vi "Load Engine Settings.vi"(8 "error in (no error)":errorcluster, 11 "Device Ref in":T1 format="%.0x") -> (0 "error out":errorcluster, 1 "FIFO Ref out":refnum<k20>, 2 "FPGA Ref out":refnum<k20>, 3 "Device Ref out":T1 format="%.0x")   [LabVIEW 2014, in "SLSC configuration Engine.lvlib"]
uses:
  SLSC configuration Engine.lvlib
  <vilib>/NI Veristand/Custom Device API/Custom Device Item Ref.ctl
  Shared/Type Defs/Device Settings.ctl
  <vilib>/NI/LVFPGA Adv Session Resources/OpenByNameSubVI.vi
  Shared/Constants.vi
  <vilib>/NI Veristand/Custom Device API/Get Item Property (Variant).vi
  <vilib>/FPGAPlugInAG/Dynamic/niLvFpga_Run_Dynamic.vi
  <vilib>/rvi/interface/common/dynamic/niFpgaEscapeDelimiterAndNull.vi
  <vilib>/Utility/error.llb/Error Cluster From Error Code.vi
  <vilib>/rvi/errors/niLvFpgaAdjustHostInterfaceError.vi
  <vilib>/rvi/interface/nirviMethod/nirviMethod.xnode
  <vilib>/NI/LVFPGA Adv Session Resources/OpenByName.xnode
  <vilib>/rvi/interface/nirviReadWriteControl/nirviReadWriteControl.xnode
  <vilib>/NI Veristand/Custom Device API/Custom Device API.lvlib
  Shared/SLSC configuration Shared.lvlib
  <vilib>/NI/LVFPGA Adv Session Resources/LVFPGAAdvSessionResources.lvlib
  NiFpgaLv.dll
  <vilib>/rvi/interface/Simulation/niFpgaSimulationCallBeginRW.vi
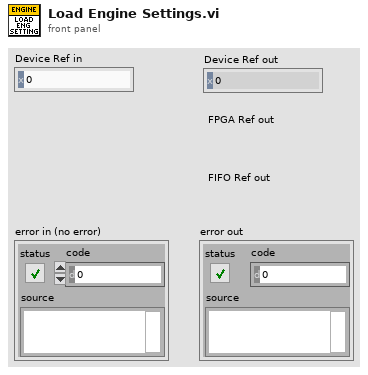
[diagram p1: front panel]
types:
  T1 = typedef "Custom Device API.lvlib/Custom Device Item Ref.ctl" = u64
  T2 = cluster{"SPI PHY Settings":cluster{"Divide Value":u8, "Transfer Length (bits)":u8, "CS Asserted Polarity":bool, "Clock Polarity (CPOL)":bool, "Clock Phase (CPHA)":bool, "Lengthen MISO Setup":bool, "Direction Change Bit":u8, "MOSI Starts as Output":bool, "Tristatable MOSI":bool}, "Sample Rate (S/s)":u32}
  T3 = cluster{"Divide Value":u8, "Transfer Length (bits)":u8, "CS Asserted Polarity":bool, "Clock Polarity (CPOL)":bool, "Clock Phase (CPHA)":bool, "Lengthen MISO Setup":bool, "Direction Change Bit":u8, "MOSI Starts as Output":bool, "Tristatable MOSI":bool}
  T4 = typedef "SLSC configuration Shared.lvlib/Device Settings.ctl" = cluster{"RIO Address":string, "Bitfile Path":path, "Load Delay (ms)":u32, "Divide Value":u8, "Sample Rate (S/s)":u32, "SLSC Settings":string, "SLSC FIFO Name":string}
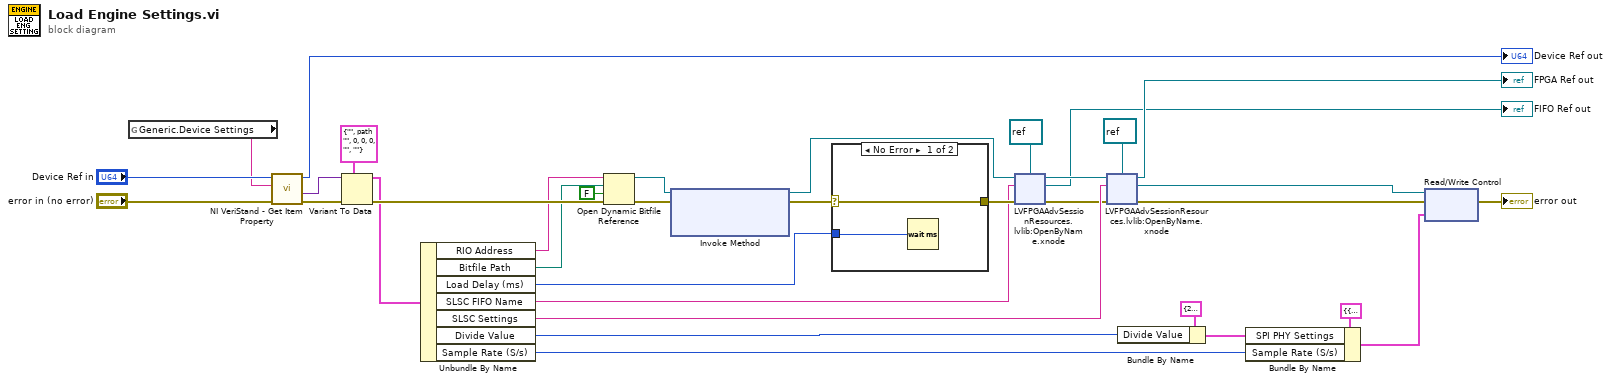
[diagram p0: block diagram]
diagram:
  n1 = global read "Constants.vi" "Generic.Device Settings"() -> (w3:string)
  n2 = call-poly <vilib>:"NI VeriStand - Get Item Property.vi"("error in (no error)"="error in (no error)", "Property Name"=w3, "Item Ref in"="Device Ref in") -> ("error out"=w11:errorcluster, "Value"=w10:variant, "Item Ref out"=→"Device Ref out":T1)  [unwired: 5 in, 1 out]
  n3 = Variant To Data(error in=w11, type=T4 {"RIO Address"="", "Bitfile Path"=path "", "Load Delay (ms)"=0, "Divide Value"=0, "Sample Rate (S/s)"=0, "SLSC Settings"="", "SLSC FIFO Name"=""} ("Cluster"), Variant=w10) -> (data=w13:T4, error out=w15:errorcluster)
  n4 = Unbundle By Name(w13) -> ("RIO Address"=w14:string, "Bitfile Path"=w2:path, "Load Delay (ms)"=w34:u32, "SLSC FIFO Name"=w30:string, "SLSC Settings"=w31:string, "Divide Value"=w21:u8, "Sample Rate (S/s)"=w27:u32)
  n5 = Open Dynamic Bitfile Reference(0:w14, 1:w2, 2:FALSE ("Run When Loaded"), 3:w15) -> (5:w7:refnum<k20>, 8:w5:errorcluster)  [unwired: 1 in]
  n6 = xnode "Invoke Method"("FPGA VI Reference In"=w7, "error in"=w5) -> ("FPGA VI Reference Out"=w8:refnum<k20>, "error out"=w32:errorcluster)  [unwired: 1 in]
  n7 = case shown="No Error" w32 {
    selector: w32 -> [w36 w38]
    tunnel: w34 -> [w37 _]
    tunnel: [w36 w38] -> w33
    frame No Error {
      n8 = Wait (ms)(milliseconds to wait=w37) -> ()  [unwired: 1 out]
    }
    frame Error {
    }
  }
  n9 = xnode "LVFPGAAdvSessionResources.lvlib:OpenByName.xnode"("FPGA VI Reference in"=w8, "Resource name in"=w30, "Single resource reference type in"=refnum<k20> refnum ("Single resource reference out"), "Error in"=w33) -> ("Single resource reference out"=→"FIFO Ref out":refnum<k20>, "Error out"=w19:errorcluster, "FPGA VI Reference out"=w22:refnum<k20>)
  n10 = xnode "LVFPGAAdvSessionResources.lvlib:OpenByName.xnode"("FPGA VI Reference in"=w22, "Resource name in"=w31, "Single resource reference type in"=refnum<k20> refnum, "Error in"=w19) -> ("Single resource reference out"=w16:refnum<k20>, "Error out"=w17:errorcluster, "FPGA VI Reference out"=→"FPGA Ref out":refnum<k20>)
  n11 = Bundle By Name(cluster=T3 {"Divide Value"=255, "Transfer Length (bits)"=32, "CS Asserted Polarity"=FALSE, "Clock Polarity (CPOL)"=FALSE, "Clock Phase (CPHA)"=FALSE, "Lengthen MISO Setup"=FALSE, "Direction Change Bit"=0, "MOSI Starts as Output"=FALSE, "Tristatable MOSI"=FALSE} ("SPI PHY Settings"), "Divide Value"=w21) -> (w26:T3)
  n12 = Bundle By Name(cluster=T2 {"SPI PHY Settings"={"Divide Value"=0, "Transfer Length (bits)"=0, "CS Asserted Polarity"=FALSE, "Clock Polarity (CPOL)"=FALSE, "Clock Phase (CPHA)"=FALSE, "Lengthen MISO Setup"=FALSE, "Direction Change Bit"=0, "MOSI Starts as Output"=FALSE, "Tristatable MOSI"=FALSE}, "Sample Rate (S/s)"=0} ("Value"), "SPI PHY Settings"=w26, "Sample Rate (S/s)"=w27) -> (w29:T2)
  n13 = xnode "Read/Write Control"("FPGA VI Reference In"=w16, "error in"=w17, "Value"=w29) -> ("error out"=→"error out":errorcluster)  [unwired: 1 out]
